vi "Space Between Buttons Write.vi"(4 "error in (no error)":errorcluster, 5 "Value":i32, 6 "Container State":T5, 7 "Display State In":T1={"Numeric"=0.0, "Array of Button References"=[], "Space Between Menu Buttons"=3, "Number of Menu Buttons"=6, "Array of Button Names"=[], "Most Recent Vertical Position"=0, "This VI"=refnum, "Current Action"=enum."Not Moving", "Most Recent Distance Traveled"=0, "Method"=enum."Resize", "Data In"=0}) -> (0 "error out":errorcluster, 3 "Display State Out":T1={"Numeric"=0.0, "Array of Button References"=[], "Space Between Menu Buttons"=3, "Number of Menu Buttons"=6, "Array of Button Names"=[], "Most Recent Vertical Position"=0, "This VI"=refnum, "Current Action"=enum."Not Moving", "Most Recent Distance Traveled"=0, "Method"=enum."Resize", "Data In"=0})   [LabVIEW 2011, in "Sliding Menu Library.lvlib" / "Sliding Menu XControl.xctl"]
uses:
  Sliding Menu XControl.xctl
  <vilib>/_xctls/Container State.ctl
  Sliding Menu State.ctl
  Menu Button Library/Menu Button xControl/Menu Button xControl.xctl
  Sliding Menu SubVIs/Sliding Menu Type Definitions/Current User Action.ctl
  Sliding Menu Methods.ctl
  Sliding Menu Data.ctl
  <vilib>/_xctls/XControlSupport.lvlib
  Sliding Menu Library.lvlib
panel:
  # "Replace the Value Control below with a Control of desired type.\nDo not remove this Control or the others from the connector pane.\nDo not change the connector pane pattern.\nThe Value control should always be the third terminal from top on the input side in the connector pane."
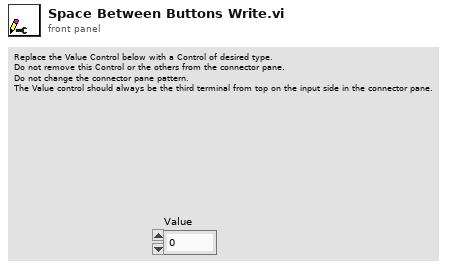
[diagram p1: front panel]
types:
  T1 = typedef "Sliding Menu Library.lvlib/Sliding Menu XControl.xctl/Sliding Menu State.ctl" = cluster{"Numeric":dbl, "Array of Button References":refnum<vi>[], "Space Between Menu Buttons":i32, "Number of Menu Buttons":i32, "Array of Button Names":string[], "Most Recent Vertical Position":i32, "This VI":refnum<vi>, "Current Action":T2, "Most Recent Distance Traveled":i32, "Method":T3, "Data In":T4}
  T2 = typedef "Sliding Menu Library.lvlib/Current User Action.ctl" = enum16{"Not Moving", "Mouse Down", "Mouse Up No Dragging", "Bounce Up Needed", "Bounce Down Needed", "Dragging", "Easing"}
  T3 = typedef "Sliding Menu Methods.ctl" = enum16{"Resize", "Move Up", "Move Down", "Move to 0"}
  T4 = typedef "Sliding Menu Library.lvlib/Sliding Menu XControl.xctl/Sliding Menu Data.ctl" = i32
  T5 = typedef "XControlSupport.lvlib/Container State.ctl" = cluster{"Indicator?":bool, "Run Mode?":bool, " Refnum":refnum<vi>}
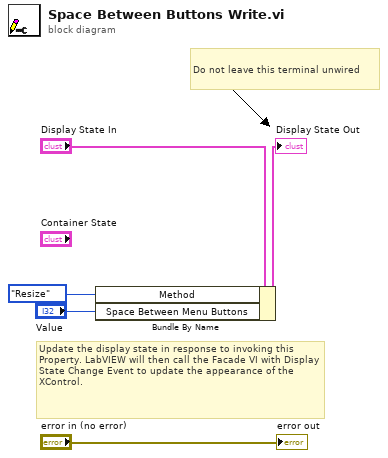
[diagram p0: block diagram]
diagram:
  # "Do not leave this terminal unwired"
  # "Update the display state in response to invoking this Property. LabVIEW will then call the Facade VI with Display State Change Event to update the appearance of the XControl."
  n1 = Bundle By Name(cluster="Display State In", "Method"=Sliding_Menu_Methods."Resize", "Space Between Menu Buttons"="Value") -> (→"Display State Out":T1)
  "error out" <- "error in (no error)"
